vi "Calculate_Compton_Edge.vi"(10 "Spectrum_Array":dbl[][](array[numeric]), 11 "Lower Cut-Off":dbl=50.0) -> (2 "Array":T1(array[cluster]), 3 "Waveform Graph":dbl[][](graph))   [LabVIEW 2019]
uses:
  SiPM_Tests_Global_Var.vi
  <vilib>/Analysis/NI_AALPro.lvlib
panel:
  in  "method":u16(ring) items=["2nd Order Central", "4th Order Central", "Forward", "Backward"]
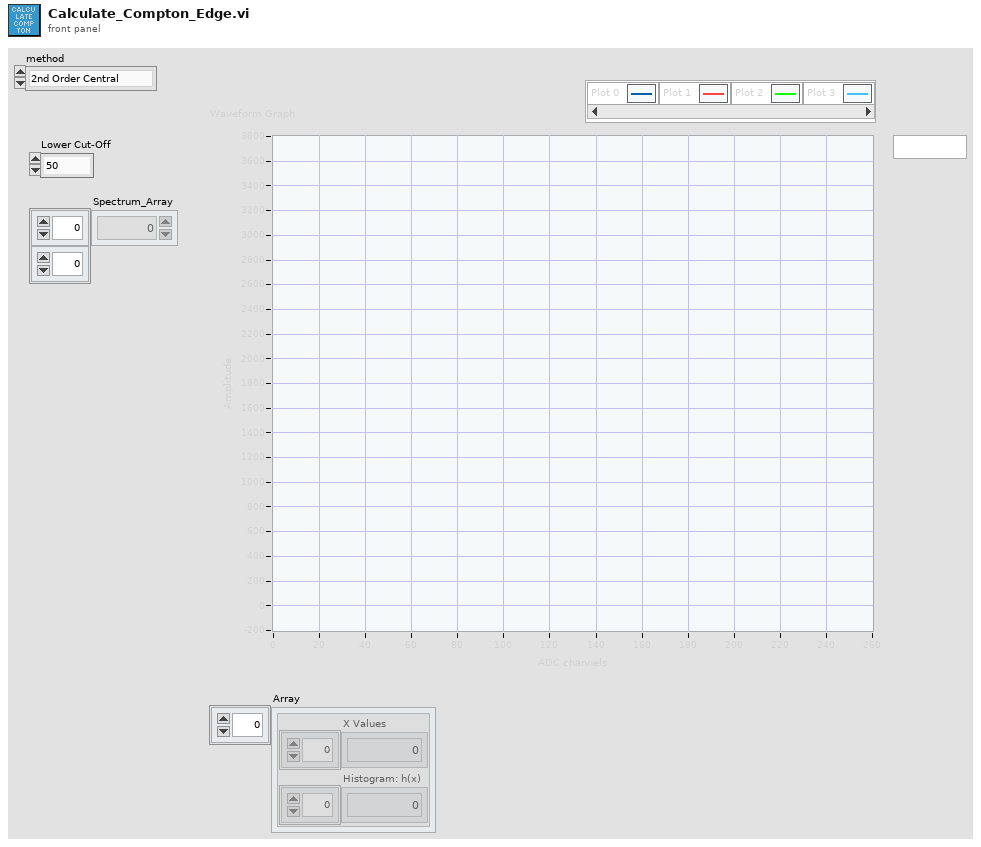
[diagram p1: front panel]
types:
  T1 = cluster{"X Values":dbl[], "Histogram: h(x)":i32[]}[]
  T2 = cluster{"X Values":dbl[], "Histogram: h(x)":i32[]}
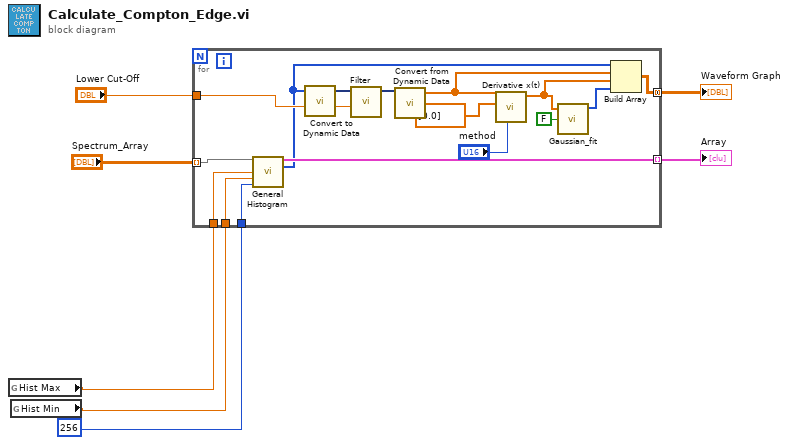
[diagram p0: block diagram]
diagram:
  n1 = global read "SiPM_Tests_Global_Var.vi" "Hist Max"() -> (w3:dbl)
  n2 = global read "SiPM_Tests_Global_Var.vi" "Hist Min"() -> (w2:dbl)
  n3 = for {
    tunnel: "Spectrum_Array" -> [w23] mode=indexing
    tunnel: w3 -> [w22]
    tunnel: w2 -> [w21]
    tunnel: 256 ("# bins") -> [w20]
    tunnel: [w19] -> w5 mode=indexing
    tunnel: [w13] -> w6 mode=concatenating
    tunnel: "Lower Cut-Off" -> [w17]
    n4 = call <vilib>:"General Histogram.vi"("X"=w23, "max"=w22, "min"=w21, "# bins"=w20) -> ("Histogram Graph"=w19:T2, "Histogram"=w12:i32[])  [unwired: 7 in, 3 out]
    n5 = call "Convert to Dynamic Data"("Array"=w12) -> ("Dynamic Data Type"=w16:dynamicdata)  [unwired: 3 in]
    n6 = call "Filter"("Lower Cut-Off"=w17, "Signal"=w16) -> ("Filtered Signal"=w15:dynamicdata)  [unwired: 8 in, 1 out]
    n7 = call "Convert from Dynamic Data"("Dynamic Data Type"=w15) -> ("Array"=w14:dbl[])  [unwired: 3 in]
    n8 = call <vilib>:"Derivative x(t).vi"("method"="method", "Initial Condition"=dbl[] [0.0], "X"=w14) -> ("dX/dt"=w10:dbl[])  [unwired: 7 in, 1 out]
    n9 = call "Gaussian_fit.vi"("Input waveform"=w10, "s"=FALSE) -> ("Gaussian fit"=w8:i32[])  [unwired: 4 in, 1 out]
    n10 = Build Array(w12, w14, w10, w8) -> (w13:dbl[][])
  }
  "Waveform Graph" <- w6
  "Array" <- w5
